vi "Q.vi"() -> ()   [LabVIEW 2013]
uses:
  dtype.ctl
panel:
  out "Array":T1[](array[typedef])
  out "x = y?":bool
  out "dt":dbl
  in  "base size":i32=10000
  in  "count":i32=100
  in  "QCnt":i32=10
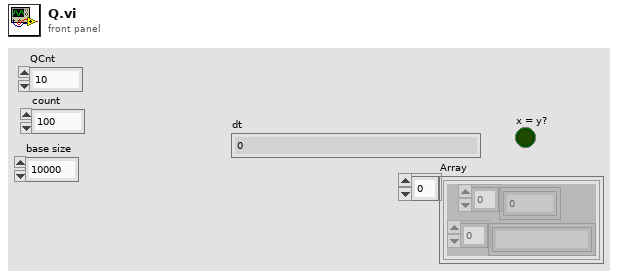
[diagram p1: front panel]
types:
  T1 = typedef "dtype.ctl" = cluster{dbl[], string[]}
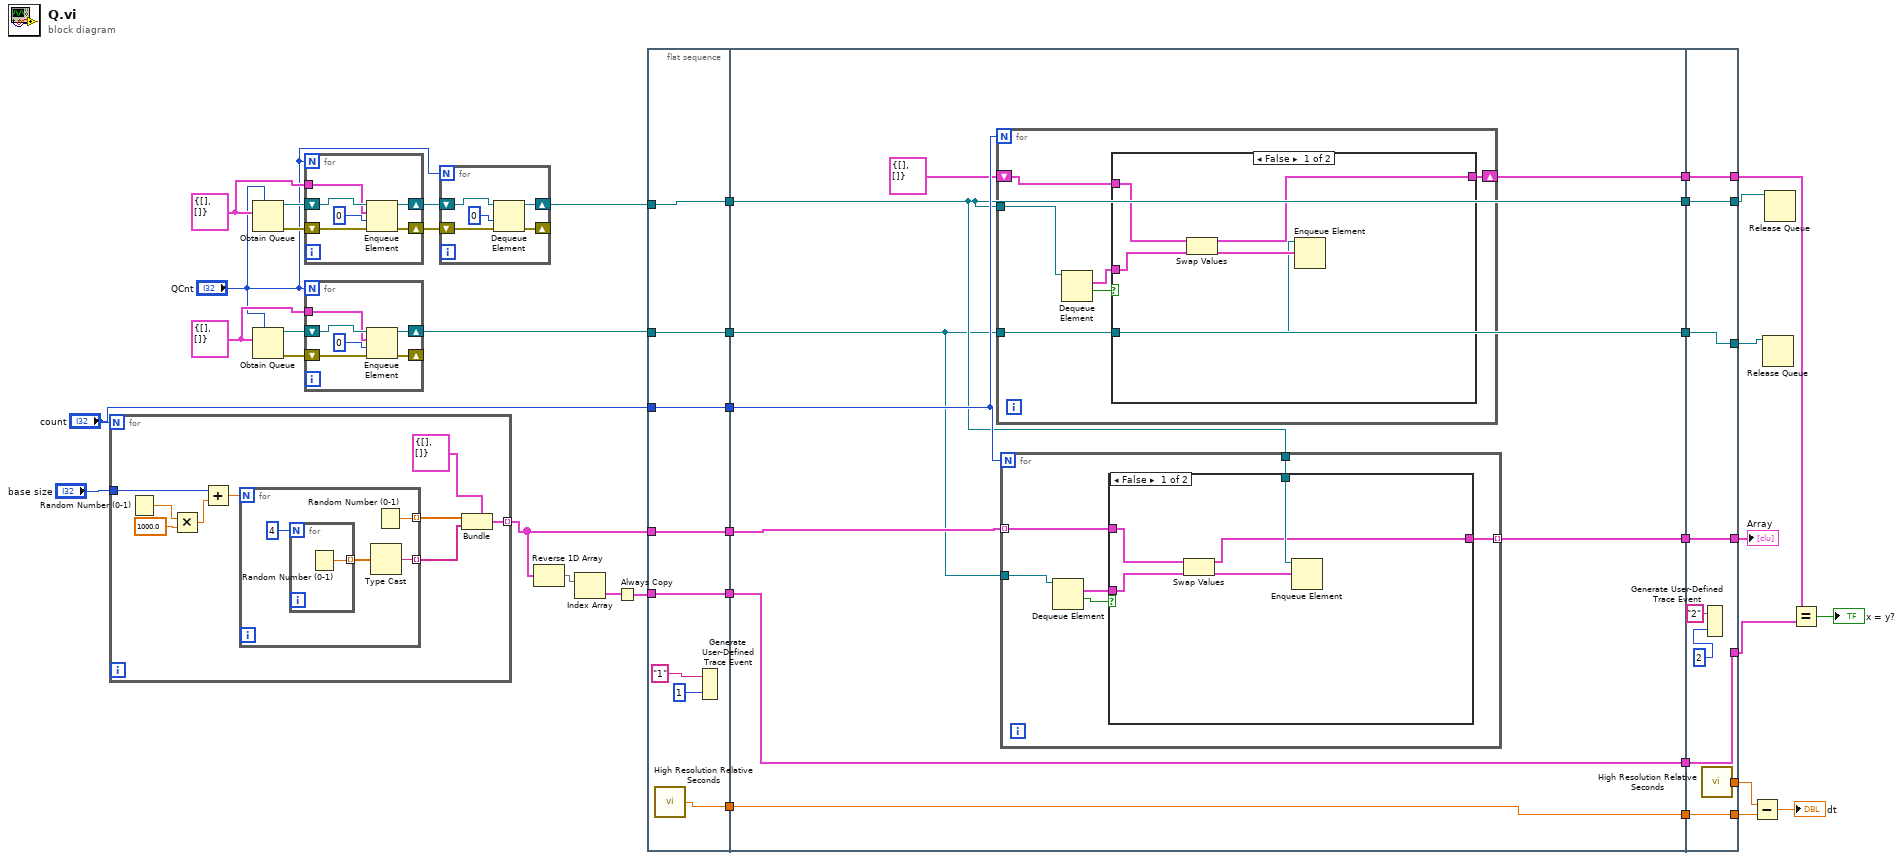
[diagram p0: block diagram]
diagram:
  w30 = T1 {[], []}
  w36 = T1 {[], []}
  n1 = for {
    N: "count" -> [_]
    tunnel: [w40] -> w11 mode=indexing
    tunnel: "base size" -> [w39]
    n2 = Random Number (0-1)() -> (number: 0 to 1=w47:dbl)
    n3 = Multiply(x=w47, y=1000.0) -> (x*y=w45:dbl)
    n4 = Add(x=w39, y=w45) -> (x+y=w44:dbl)
    n5 = for {
      N: w44 -> [_]
      tunnel: [w51] -> w42 mode=indexing
      tunnel: [w48] -> w41 mode=indexing
      n6 = for {
        N: 4 -> [_]
        tunnel: [w52] -> w49 mode=indexing
        n7 = Random Number (0-1)() -> (number: 0 to 1=w52:dbl)
      }
      n8 = Type Cast(x=w49) -> (*(type *) &x=w48:string)  [unwired: 1 in]
      n9 = Random Number (0-1)() -> (number: 0 to 1=w51:dbl)
    }
    n10 = Bundle(cluster=T1 {[], []}, w42, w41) -> (w40:T1)
  }
  n11 = Obtain Queue(max queue size (-1, unlimited)="QCnt", element data type=w36) -> (queue out=w37:refnum<queue>, error out=w33:errorcluster)  [unwired: 3 in, 1 out]
  n12 = Obtain Queue(max queue size (-1, unlimited)="QCnt", element data type=w30) -> (queue out=w29:refnum<queue>, error out=w32:errorcluster)  [unwired: 3 in, 1 out]
  n13 = for {
    N: "QCnt" -> [_]
    shift-right: [w57] -> w35
    shift-left: w37 -> [w58]
    tunnel: w36 -> [w56]
    shift-right: [w54] -> w34
    shift-left: w33 -> [w53]
    n14 = Enqueue Element(queue=w58, element=w56, timeout in ms (-1)=0, error in (no error)=w53) -> (queue out=w57:refnum<queue>, error out=w54:errorcluster)  [unwired: 1 out]
  }
  n15 = for {
    N: "QCnt" -> [_]
    shift-right: [w63] -> w31
    shift-left: w29 -> [w64]
    tunnel: w30 -> [w62]
    shift-right: [w60] -> _
    shift-left: w32 -> [w59]
    n16 = Enqueue Element(queue=w64, element=w62, timeout in ms (-1)=0, error in (no error)=w59) -> (queue out=w63:refnum<queue>, error out=w60:errorcluster)  [unwired: 1 out]
  }
  n17 = for {
    N: "QCnt" -> [_]
    shift-right: [w68] -> w21
    shift-left: w35 -> [w69]
    shift-right: [w66] -> _
    shift-left: w34 -> [w67]
    n18 = Dequeue Element(queue=w69, timeout in ms (-1)=0, error in (no error)=w67) -> (queue out=w68:refnum<queue>, error out=w66:errorcluster)  [unwired: 2 out]
  }
  n19 = Reverse 1D Array(array=w11) -> (reversed array=w12:T1[])
  n20 = Index Array(array=w12) -> (element=w10:T1)  [unwired: 1 in]
  n21 = Always Copy(1:w10) -> (0:w7:T1)
  n22 = flat-sequence {
    tunnel: [w77] -> w27
    tunnel: [w76] -> w22
    tunnel: w21 -> [w76]
    tunnel: [w75] -> w19
    tunnel: w31 -> [w75]
    tunnel: [w74] -> w16
    tunnel: "count" -> [w74]
    tunnel: [w73] -> w14
    tunnel: w11 -> [w73]
    tunnel: [w72] -> w8
    tunnel: w7 -> [w72]
    tunnel: w27 -> [w86]
    tunnel: [w86] -> w26
    tunnel: [w83] -> w23
    tunnel: w22 -> [w83]
    tunnel: [w81] -> w20
    tunnel: w19 -> [w81]
    tunnel: w16 -> [w85]
    tunnel: w14 -> [w84]
    tunnel: [w80] -> w13
    tunnel: [w79] -> w9
    tunnel: w8 -> [w79]
    tunnel: [w78] -> w2
    tunnel: [w119] -> w28
    tunnel: w26 -> [w118]
    tunnel: [w118] -> w25
    tunnel: [w117] -> w18
    tunnel: w23 -> [w117]
    tunnel: [w116] -> w17
    tunnel: w20 -> [w116]
    tunnel: [w115] -> w5
    tunnel: w13 -> [w115]
    tunnel: [w114] -> w6
    tunnel: w9 -> [w114]
    tunnel: [w111] -> w1
    tunnel: w2 -> [w111]
    frame #0 {
      n23 = call <vilib>:"High Resolution Relative Seconds.vi"() -> ("relative seconds"=w77:dbl)
      n24 = Generate User-Defined Trace Event(1:1 ("trace integer"), 2:"1" ("trace string")) -> ()
    }
    frame #1 {
      n25 = for {
        N: w85 -> [_]
        tunnel: w83 -> [w104]
        shift-right: [w101] -> w80
        shift-left: T1 {[], []} -> [w102]
        tunnel: w81 -> [w99]
        n26 = Dequeue Element(queue=w104) -> (element=w100:T1, timed out?=w103:bool)  [unwired: 2 in, 2 out]
        n27 = case shown="False" w103 {
          tunnel: w100 -> [w109 _]
          tunnel: w102 -> [w107 w110]
          tunnel: [w105 w110] -> w101
          tunnel: w99 -> [w106 _]
          frame False {
            n28 = Swap Values(12:w107, 14:w109) -> (1:w105:T1, 3:w108:T1)  [unwired: 1 in]
            n29 = Enqueue Element(queue=w106, element=w108) -> ()  [unwired: 2 in, 3 out]
          }
          frame True {
          }
        }
      }
      n30 = for {
        N: w85 -> [_]
        tunnel: w84 -> [w89] mode=indexing
        tunnel: w81 -> [w92]
        tunnel: w83 -> [w88]
        tunnel: [w87] -> w78 mode=indexing
        n31 = Dequeue Element(queue=w92) -> (element=w90:T1, timed out?=w91:bool)  [unwired: 2 in, 2 out]
        n32 = case shown="False" w91 {
          tunnel: w90 -> [w97 _]
          tunnel: w89 -> [w96 w98]
          tunnel: w88 -> [w95 _]
          tunnel: [w93 w98] -> w87
          frame False {
            n33 = Swap Values(12:w96, 14:w97) -> (1:w93:T1, 3:w94:T1)  [unwired: 1 in]
            n34 = Enqueue Element(queue=w95, element=w94) -> ()  [unwired: 2 in, 3 out]
          }
          frame True {
          }
        }
      }
    }
    frame #2 {
      n35 = Generate User-Defined Trace Event(1:2 ("trace integer"), 2:"2" ("trace string")) -> ()
      n36 = call <vilib>:"High Resolution Relative Seconds.vi"() -> ("relative seconds"=w119:dbl)
    }
  }
  n37 = Subtract(x=w28, y=w25) -> (x-y=→"dt":dbl)
  n38 = Release Queue(queue=w17) -> ()  [unwired: 2 in, 3 out]
  n39 = Release Queue(queue=w18) -> ()  [unwired: 2 in, 3 out]
  n40 = Equal?(x=w5, y=w6) -> (x = y?=→"x = y?":bool)
  "Array" <- w1
